vi "Main.vi"(0 "Operation":string(combo)="Add", 1 "Delete":bool, 5 "Add":bool, 7 "Load":bool, 9 "Save":bool, 11 "Error In":errorcluster, 12 "Tree":string(tree)) -> (15 "Error Out":errorcluster)   [LabVIEW 2021, in "Calculator.lvlib"]
doc: "This VI acts as a calculator , which has four child classes with the overriding methods and seperate UI VIs for each class which is opened in subpanel when the particular instance is selected. Also the class data is stored in XML file and it can be loaded when required."
uses:
  Calculator.lvlib
  Controls/Queue Operations.ctl
  Classes/NumericOperation/NumericOperation.lvclass
  Controls/Data Cluster.ctl
  Controls/Class Data.ctl
  Controls/User Event Operations.ctl
  <vilib>/Utility/xml.llb/Write to XML File(string).vi
  <vilib>/Utility/xml.llb/Read From XML File(array).vi
panel:
  in  "Help Button":bool
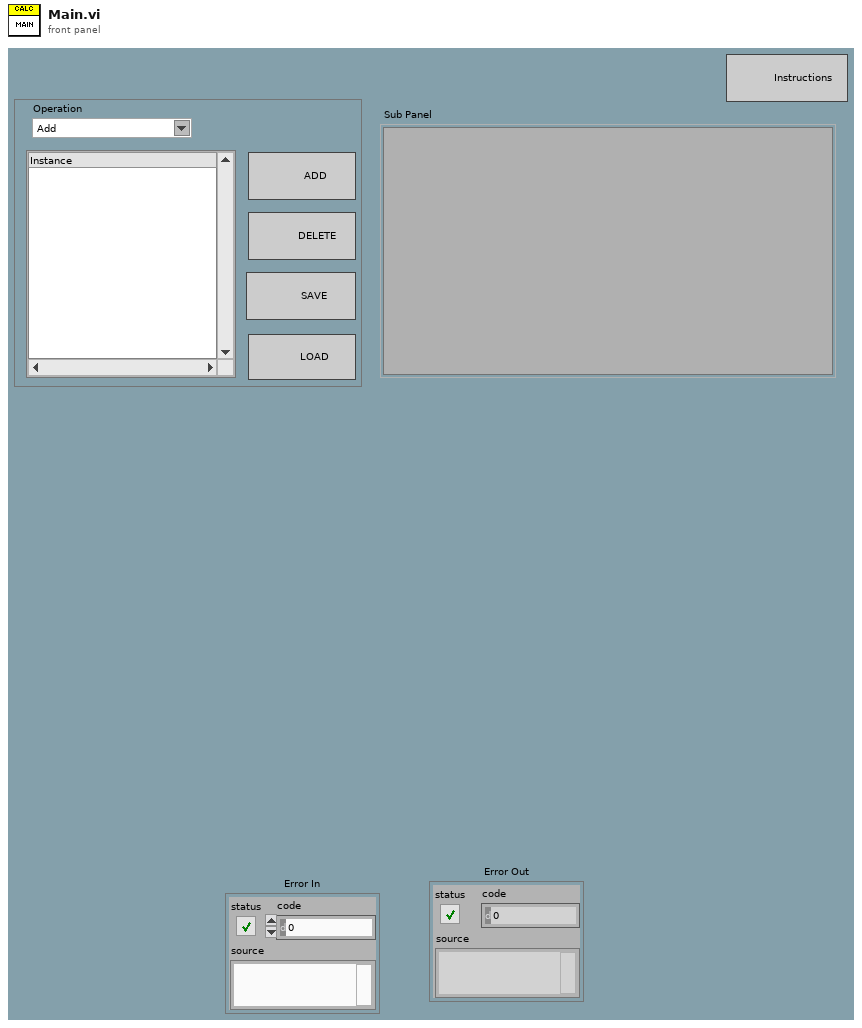
[diagram p1: front panel]
types:
  T1 = typedef "Calculator.lvlib/User Event Operations.ctl" = enum16{"Obtain", "Generate", "Release"}
  T2 = typedef "Calculator.lvlib/Queue Operations.ctl" = enum16{"Create", "Enqueue", "EnqueueN", "Enqueue at top", "Dequeue", "Flush", "Release"}
  T3 = typedef "Calculator.lvlib/Data Cluster.ctl" = cluster{"A":dbl, "B":dbl, "C":dbl, "NumericOperation.lvclass":refnum<class "NumericOperation.lvclass">, "generic class reference":refnum<class "NumericOperation.lvclass">, "Operation":string, "Active Tag":string, "Path":path, "VI Refnum":refnum<vi>, "Class Data":refnum<class "NumericOperation.lvclass">, "DataArray":T4[], "FilePath":path, "Class Name":string, "Data Value Reference Out":refnum<data-value>}
  T4 = typedef "Calculator.lvlib/Class Data.ctl" = cluster{"Class Data":refnum<class "NumericOperation.lvclass">, "String":string}
  T5 = typedef "LVPoint32TypeDef.ctl" = cluster{"Horizontal":i32, "Vertical":i32}
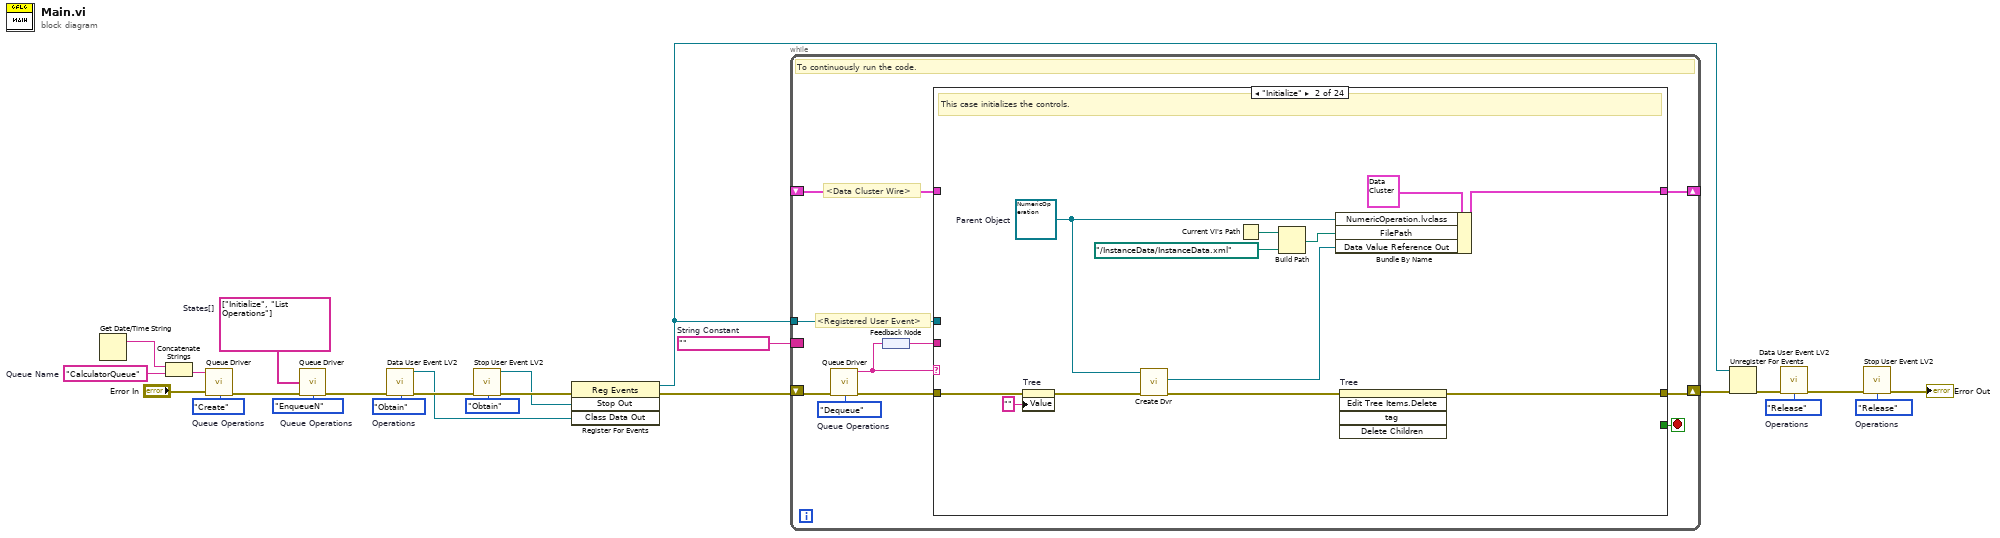
[diagram p0: block diagram]
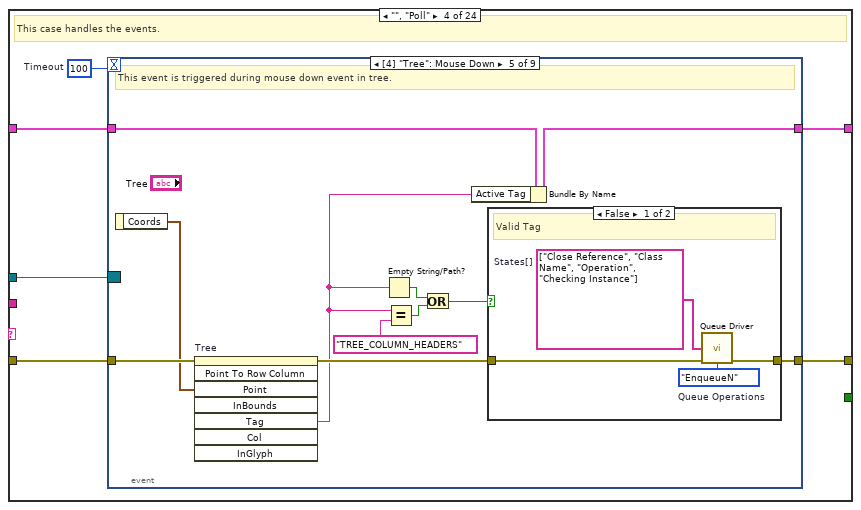
[diagram p4: hidden frame]
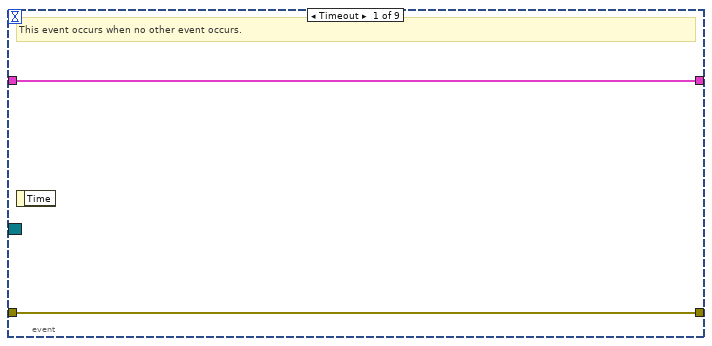
[diagram p5: hidden frame]
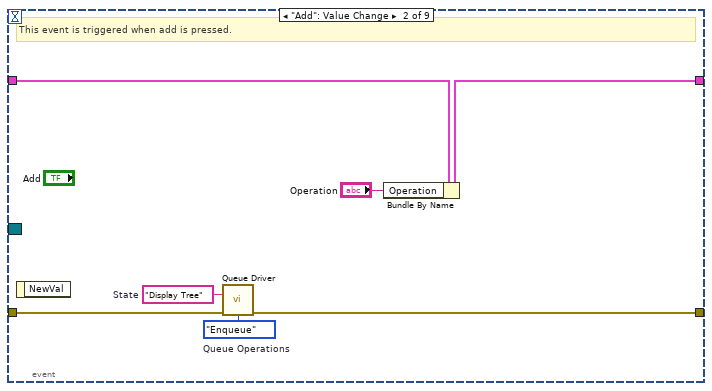
[diagram p6: hidden frame]
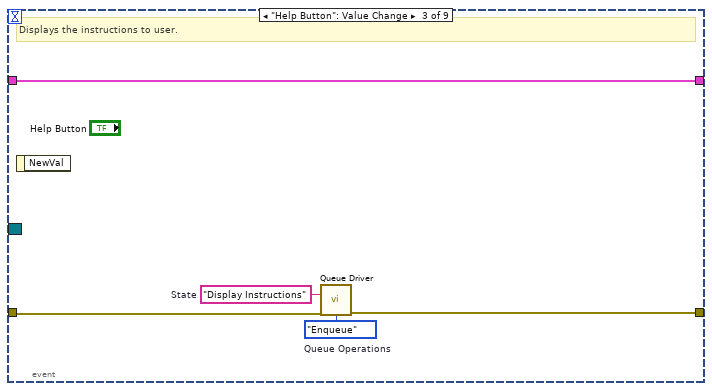
[diagram p7: hidden frame]
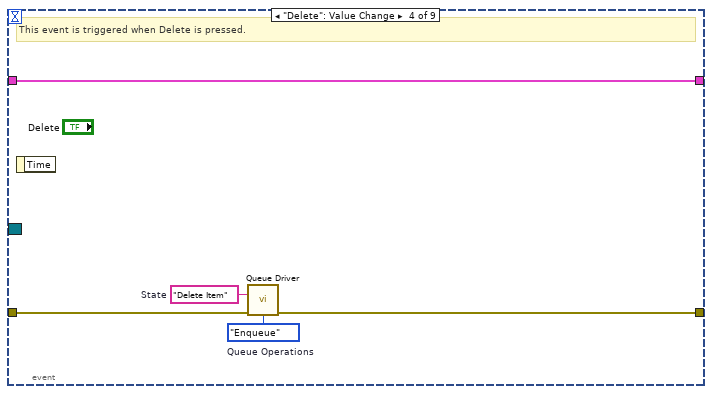
[diagram p8: hidden frame]
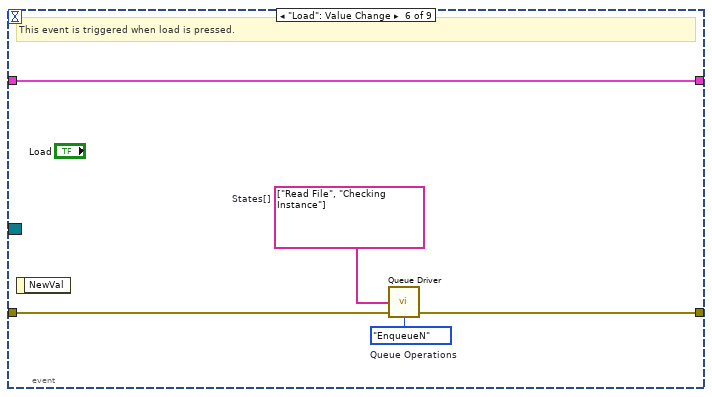
[diagram p10: hidden frame]
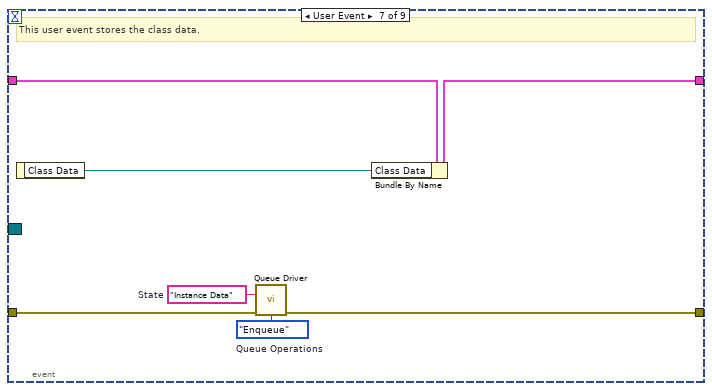
[diagram p11: hidden frame]
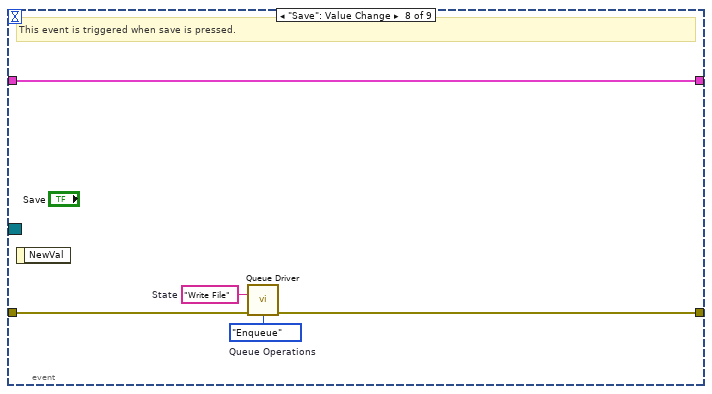
[diagram p12: hidden frame]
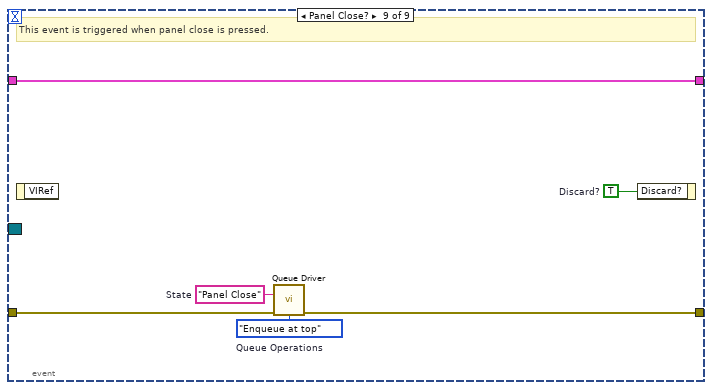
[diagram p13: hidden frame]
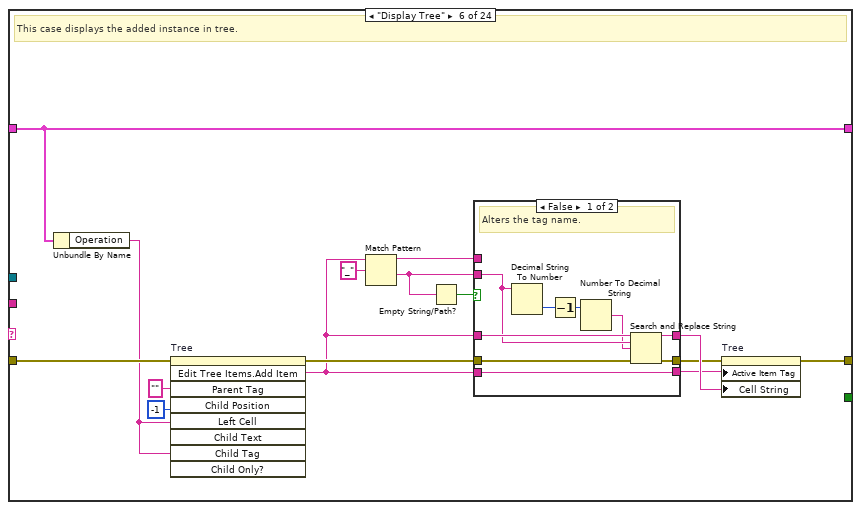
[diagram p15: hidden frame]
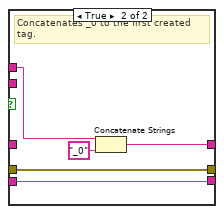
[diagram p16: hidden frame]
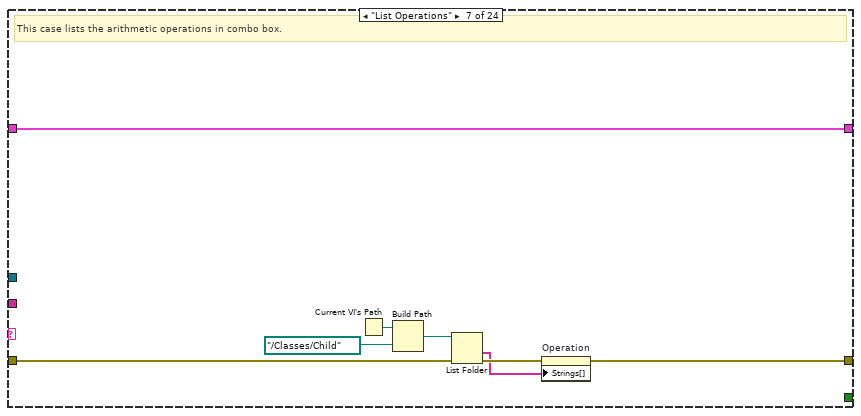
[diagram p17: hidden frame]
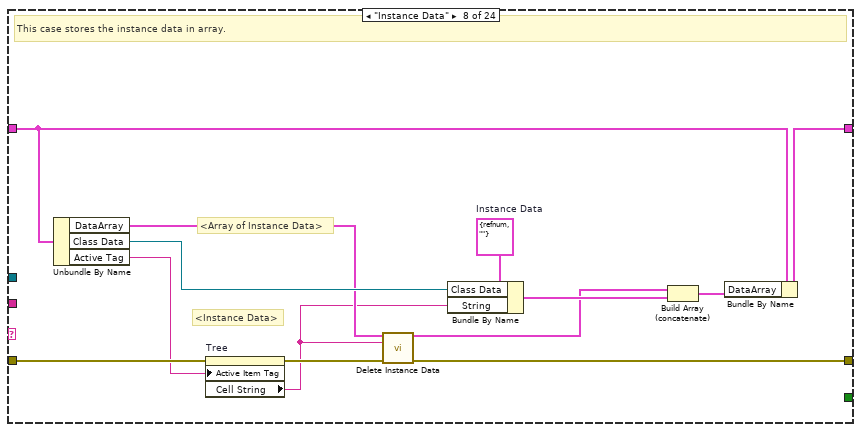
[diagram p18: hidden frame]
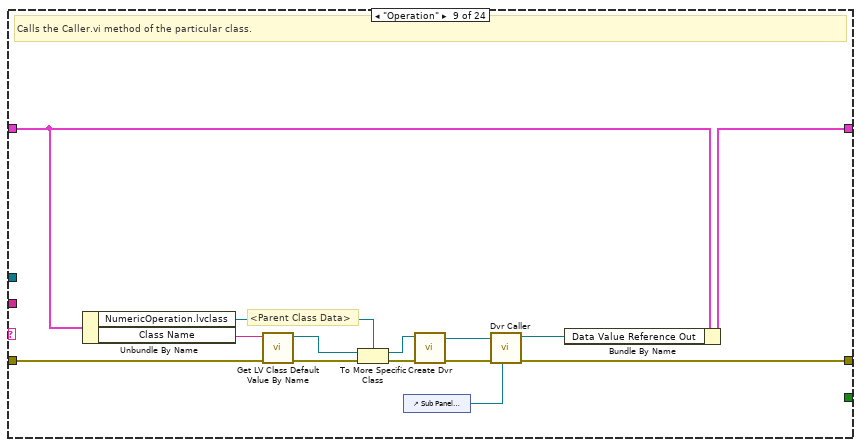
[diagram p19: hidden frame]
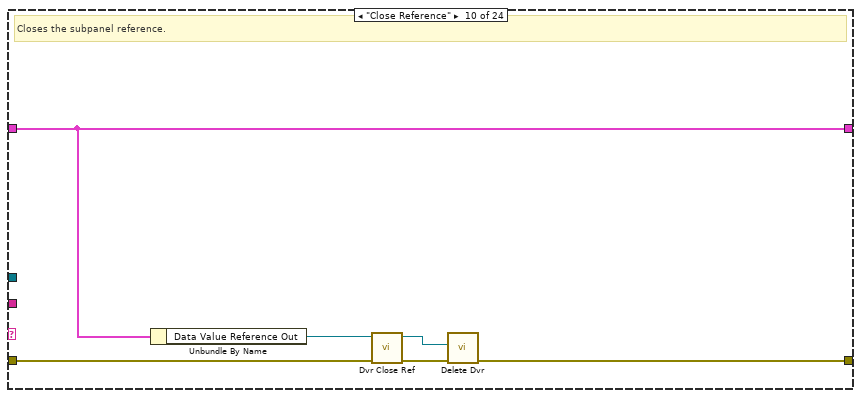
[diagram p20: hidden frame]
diagram:
  w1 = string[] ["Initialize", "List Operations"]  # States[]
  w2 = ""  # String Constant
  w3 = User_Event_Operations."Release"  # Operations
  w4 = User_Event_Operations."Release"  # Operations
  w11 = User_Event_Operations."Obtain"  # Operations
  w21 = Queue_Operations."EnqueueN"  # Queue Operations
  w19 = "CalculatorQueue"  # Queue Name
  w23 = Queue_Operations."Create"  # Queue Operations
  n1 = Get Date/Time String() -> (date string=w20:string)  [unwired: 3 in, 1 out]
  n2 = Concatenate Strings(w20, w19) -> (w18:string)
  n3 = call "Queue Driver.vi"("Queue Name"=w18, "Error In"="Error In", "Queue Operations"=w23) -> ("Error Out"=w22:errorcluster)  [unwired: 11 in, 1 out]
  n4 = call "Queue Driver.vi"("States[]"=w1, "Error In"=w22, "Queue Operations"=w21) -> ("Error Out"=w13:errorcluster)  [unwired: 11 in, 1 out]
  n5 = call "Data User Event LV2.vi"("Error In"=w13, "Operations"=w11) -> ("Class Data Out"=w8:refnum<user-event>, "Error Out"=w14:errorcluster)  [unwired: 12 in]
  n6 = call "Stop User Event LV2.vi"("Error In"=w14, "Operations"=User_Event_Operations."Obtain") -> ("Stop Out"=w9:refnum<user-event>, "Error Out"=w12:errorcluster)  [unwired: 12 in]
  n7 = register-events(error in=w12, w9, w8) -> (reference out=w15:refnum<event-registration>, error out=w17:errorcluster)  [unwired: 1 in]
  n8 = while {
    shift-right: [w32] -> _
    shift-left: _ -> [w33]
    shift-right: [w29] -> w16
    shift-left: w17 -> [w30]
    border: w2 -> [_]
    tunnel: w15 -> [w25]
    stop <- w26 stop-if-true
    w34 = Queue_Operations."Dequeue"  # Queue Operations
    # "<Registered User Event>"
    # "<Data Cluster Wire>"
    # "To continuously run the code."
    n9 = call "Queue Driver.vi"("Error In"=w30, "Queue Operations"=w34) -> ("Dequeued Element"=w28:string, "Error Out"=w31:errorcluster)  [unwired: 12 in]
    n10 = feedback-in #1(w28) -> ()
    n11 = feedback #1() -> (w27:string)
    n12 = case shown="\"Initialize\"" w28 {
      tunnel: w33 -> [w36 _ w50 w55 w116 w122 w153 w165 w175 w186 w190 w218 w226 w247 w256 w262 w276 w292 w297 w304 w307 w309 w312 w329]
      tunnel: [w36 w48 w50 w54 w116 w122 w153 w164 w177 w186 w188 w217 w226 w247 w256 w262 w275 w292 w297 w304 w307 w309 w312 w329] -> w32
      tunnel: w31 -> [w35 w39 w49 w53 w115 w131 w149 w166 w176 w185 w194 w216 w221 w246 w255 w259 w280 w291 w296 w303 w306 w308 w311 w328]
      tunnel: [w35 w46 w49 w52 w115 w126 w152 w157 w171 w182 w195 w216 w224 w245 w255 w260 w273 w291 w299 w303 w306 w308 w314 w328] -> w29
      tunnel: w27 -> [_ _ _ _ _ _ _ _ _ _ _ _ _ _ _ _ _ _ _ _ _ _ w321 _]
      tunnel: [_ _ _ _ _ _ _ _ _ _ _ _ _ _ _ _ _ _ w298 _ _ _ _ _] -> w26
      tunnel: w25 -> [_ _ _ w51 _ _ _ _ _ _ _ _ _ _ _ _ _ _ _ _ _ _ _ _]
      frame "/******** Initializing********/" {
        # "Splitter case for initialization."
      }
      frame "Initialize" {
        w41 = refnum<class "NumericOperation.lvclass"> refnum  # Parent Object
        # "This case initializes the controls."
        n13 = property on="Tree" class="Tree (strict)"(error in=w39, "Value"="" ("Tree")) -> (error out=w38:errorcluster)  [unwired: 1 in, 1 out]
        n14 = call "Create Dvr.vi"("Error In"=w38, "NumericOperation in"=w41) -> ("Error Out"=w42:errorcluster, "Data Value Reference"=w40:refnum<data-value>)  [unwired: 7 in, 1 out]
        n15 = Current VI's Path() -> (path=w45:path)
        n16 = Build Path(base path=w45, name or relative path=path "../InstanceData/InstanceData.xml") -> (appended path=w47:path)
        n17 = Bundle By Name(cluster=T3 {"A"=0.0, "B"=0.0, "C"=0.0, "NumericOperation.lvclass"=refnum, "generic class reference"=refnum, "Operation"="", "Active Tag"="", "Path"=path "", "VI Refnum"=refnum, "Class Data"=refnum, "DataArray"=[], "FilePath"=path "", "Class Name"="", "Data Value Reference Out"=refnum}, "NumericOperation.lvclass"=w41, "FilePath"=w47, "Data Value Reference Out"=w40) -> (w48:T3)
        n18 = invoke on="Tree" class="Tree (strict)" method="Edit Tree Items.Delete"(error in=w42) -> (error out=w46:errorcluster)  [unwired: 4 in, 4 out]
      }
      frame "/******** Poll ********/" {
        # "Splitter case for poll."
      }
      frame "", "Poll" {
        w56 = 100  # Timeout
        # "This case handles the events."
        n19 = event shown="[4] \"Tree\": Mouse Down" {
          selector: w51 -> [_ _ _ _ _ _ _ _ _]
          dyn-events: _ -> [_ _ _ _ _ _ _ _ _]
          timeout: w56 -> [_ _ _ _ _ _ _ _ _]
          tunnel: w55 -> [w58 w61 w66 w71 w84 w96 w103 w108 w111]
          tunnel: [w58 w60 w66 w71 w83 w96 w101 w108 w111] -> w54
          tunnel: w53 -> [w57 w65 w70 w75 w86 w94 w99 w107 w114]
          tunnel: [w57 w64 w69 w74 w81 w95 w100 w106 w113] -> w52
          event Timeout {
            # "This event occurs when no other event occurs."
            n20 = event-data() -> ()  [unwired: 1 in, 1 out]
          }
          event "Add": Value Change {
            w62 = "Display Tree"  # State
            w63 = Queue_Operations."Enqueue"  # Queue Operations
            # "This event is triggered when add is pressed."
            n21 = event-data() -> ()  [unwired: 1 in, 1 out]
            n22 = call "Queue Driver.vi"("State"=w62, "Error In"=w65, "Queue Operations"=w63) -> ("Error Out"=w64:errorcluster)  [unwired: 11 in, 1 out]
            n23 = Bundle By Name(cluster=w61, "Operation"="Operation") -> (w60:T3)
          }
          event "Help Button": Value Change {
            w67 = "Display Instructions"  # State
            w68 = Queue_Operations."Enqueue"  # Queue Operations
            # "Displays the instructions to user."
            n24 = event-data() -> ()  [unwired: 1 in, 1 out]
            n25 = call "Queue Driver.vi"("State"=w67, "Error In"=w70, "Queue Operations"=w68) -> ("Error Out"=w69:errorcluster)  [unwired: 11 in, 1 out]
          }
          event "Delete": Value Change {
            w72 = "Delete Item"  # State
            w73 = Queue_Operations."Enqueue"  # Queue Operations
            # "This event is triggered when Delete is pressed."
            n26 = event-data() -> ()  [unwired: 1 in, 1 out]
            n27 = call "Queue Driver.vi"("State"=w72, "Error In"=w75, "Queue Operations"=w73) -> ("Error Out"=w74:errorcluster)  [unwired: 11 in, 1 out]
          }
          event "Tree": Mouse Down {
            # "This event is triggered during mouse down event in tree."
            n28 = event-data() -> ("Coords"=w85:T5)  [unwired: 1 in]
            n29 = invoke on="Tree" class="Tree (strict)" method="Point To Row Column"(error in=w86, "Point"=w85) -> (error out=w82:errorcluster, "Tag"=w80:string)  [unwired: 6 in, 6 out]
            n30 = Empty String/Path?(string/path=w80) -> (empty?=w77:bool)
            n31 = Equal?(x=w80, y="TREE_COLUMN_HEADERS") -> (x = y?=w78:bool)
            n32 = Or(x=w77, y=w78) -> (x .or. y?=w76:bool)
            n33 = Bundle By Name(cluster=w84, "Active Tag"=w80) -> (w83:T3)
            n34 = case shown="False" w76 {
              tunnel: w82 -> [w90 w91]
              tunnel: [w89 w91] -> w81
              frame False {
                w87 = string[] ["Close Reference", "Class Name", "Operation", "Checking Instance"]  # States[]
                w88 = Queue_Operations."EnqueueN"  # Queue Operations
                # "Valid Tag"
                n35 = call "Queue Driver.vi"("States[]"=w87, "Error In"=w90, "Queue Operations"=w88) -> ("Error Out"=w89:errorcluster)  [unwired: 11 in, 1 out]
              }
              frame True {
                # "Invalid Tag"
              }
            }
          }
          event "Load": Value Change {
            w92 = string[] ["Read File", "Checking Instance"]  # States[]
            w93 = Queue_Operations."EnqueueN"  # Queue Operations
            # "This event is triggered when load is pressed."
            n36 = event-data() -> ()  [unwired: 1 in, 1 out]
            n37 = call "Queue Driver.vi"("States[]"=w92, "Error In"=w94, "Queue Operations"=w93) -> ("Error Out"=w95:errorcluster)  [unwired: 11 in, 1 out]
          }
          event User Event {
            w97 = "Instance Data"  # State
            w98 = Queue_Operations."Enqueue"  # Queue Operations
            # "This user event stores the class data."
            n38 = event-data() -> ("Class Data"=w102:refnum<class "NumericOperation.lvclass">)  [unwired: 1 in]
            n39 = call "Queue Driver.vi"("State"=w97, "Error In"=w99, "Queue Operations"=w98) -> ("Error Out"=w100:errorcluster)  [unwired: 11 in, 1 out]
            n40 = Bundle By Name(cluster=w103, "Class Data"=w102) -> (w101:T3)
          }
          event "Save": Value Change {
            w104 = "Write File"  # State
            w105 = Queue_Operations."Enqueue"  # Queue Operations
            # "This event is triggered when save is pressed."
            n41 = event-data() -> ()  [unwired: 1 in, 1 out]
            n42 = call "Queue Driver.vi"("State"=w104, "Error In"=w107, "Queue Operations"=w105) -> ("Error Out"=w106:errorcluster)  [unwired: 11 in, 1 out]
          }
          event Panel Close? {
            w110 = Queue_Operations."Enqueue at top"  # Queue Operations
            w112 = "Panel Close"  # State
            w109 = TRUE  # Discard?
            # "This event is triggered when panel close is pressed."
            n43 = event-data() -> ()  [unwired: 1 in, 1 out]
            n44 = call "Queue Driver.vi"("State"=w112, "Error In"=w114, "Queue Operations"=w110) -> ("Error Out"=w113:errorcluster)  [unwired: 11 in, 1 out]
            n45 = event-data("Discard?"=w109) -> ()  [unwired: 1 in, 1 out]
          }
        }
      }
      frame "/******** Functionalities ********/" {
        # "Splitter case for functionalities."
      }
      frame "Display Tree" {
        # "This case displays the added instance in tree."
        n46 = Unbundle By Name(w122) -> ("Operation"=w121:string)
        n47 = invoke on="Tree" class="Tree (strict)" method="Edit Tree Items.Add Item"(error in=w131, "Parent Tag"="", "Child Position"=-1, "Left Cell"=w121, "Child Tag"=w121) -> (error out=w120:errorcluster, "Edit Tree Items:Add Item"=w118:string)  [unwired: 4 in, 7 out]
        n48 = Match Pattern(string=w118, regular expression="_") -> (before substring=w127:string, after substring=w123:string)  [unwired: 1 in, 2 out]
        n49 = Empty String/Path?(string/path=w123) -> (empty?=w124:bool)
        n50 = case shown="False" w124 {
          tunnel: [w137 w144] -> w125
          tunnel: w127 -> [_ w143]
          tunnel: w123 -> [w138 _]
          tunnel: w118 -> [w139 _]
          tunnel: w120 -> [w134 w142]
          tunnel: [w133 w142] -> w119
          tunnel: [w132 w141] -> w117
          tunnel: w118 -> [w132 w141]
          frame False {
            # "Alters the tag name."
            n51 = Decimal String To Number(string=w138) -> (number=w136:i32)  [unwired: 2 in, 1 out]
            n52 = Decrement(x=w136) -> (x-1=w140:i32)
            n53 = Number To Decimal String(number=w140) -> (decimal integer string=w135:string)  [unwired: 1 in]
            n54 = Search and Replace String(input string=w139, search string=w138, replace string=w135, error in=w134) -> (result string=w137:string, error out=w133:errorcluster)  [unwired: 4 in, 2 out]
          }
          frame True {
            # "Concatenates _0 to the first created tag."
            n55 = Concatenate Strings(w143, "_0" ("string")) -> (w144:string)
          }
        }
        n56 = property on="Tree" class="Tree (strict)"(error in=w119, "Active Item Tag"=w117, "Cell String"=w125) -> (error out=w126:errorcluster)  [unwired: 1 in, 1 out]
      }
      frame "List Operations" {
        # "This case lists the arithmetic operations in combo box."
        n57 = Current VI's Path() -> (path=w151:path)
        n58 = Build Path(base path=w151, name or relative path=path "../Classes/Child") -> (appended path=w147:path)
        n59 = List Folder(path=w147, error in=w149) -> (folder names=w146:string[], error out=w148:errorcluster)  [unwired: 2 in, 2 out]
        n60 = property on="Operation" class="CmbBox"(error in=w148, "Strings[]"=w146) -> (error out=w152:errorcluster)  [unwired: 1 in, 1 out]
      }
      frame "Instance Data" {
        w162 = T4 {"Class Data"=refnum, "String"=""}  # Instance Data
        # "<Array of Instance Data>"
        # "<Instance Data>"
        # "This case stores the instance data in array."
        n61 = Unbundle By Name(w165) -> ("DataArray"=w156:T4[], "Class Data"=w161:refnum<class "NumericOperation.lvclass">, "Active Tag"=w163:string)
        n62 = property on="Tree" class="Tree (strict)"(error in=w166, "Active Item Tag"=w163) -> (error out=w158:errorcluster, "Cell String"=w155:string)  [unwired: 1 in, 1 out]
        n63 = call "Delete Instance Data.vi"("Data Array"=w156, "Cell String"=w155, "Error In"=w158) -> ("Data Array Out"=w154:T4[], "Error Out"=w157:errorcluster)  [unwired: 11 in]
        n64 = Bundle By Name(cluster=w162, "Class Data"=w161, "String"=w155) -> (w160:T4)
        n65 = Build Array (concatenate)(w154, w160) -> (w159:T4[])
        n66 = Bundle By Name(cluster=w165, "DataArray"=w159) -> (w164:T3)
      }
      frame "Operation" {
        # "<Parent Class Data>"
        # "Calls the Caller.vi method of the particular class."
        n67 = Unbundle By Name(w175) -> ("NumericOperation.lvclass"=w174:refnum<class "NumericOperation.lvclass">, "Class Name"=w178:string)
        n68 = call <vilib>:"Get LV Class Default Value By Name.vi"("error in (no error)"=w176, "class name"=w178) -> ("error out"=w179:errorcluster, "object"=w180:refnum<class>)  [unwired: 8 in]
        n69 = To More Specific Class(target class=w174, reference=w180, error in=w179) -> (specific class reference=w170:refnum<class "NumericOperation.lvclass">, error out=w172:errorcluster)
        n70 = control-ref of="Sub Panel Reference"() -> (w168:refnum<vi>)
        n71 = call "Create Dvr.vi"("Error In"=w172, "NumericOperation in"=w170) -> ("Error Out"=w173:errorcluster, "Data Value Reference"=w169:refnum<data-value>)  [unwired: 7 in, 1 out]
        n72 = call "Dvr Caller.vi"("Sub Panel"=w168, "Error In"=w173, "Data Value Reference In"=w169) -> ("Error Out"=w171:errorcluster, "Data Value Reference Out"=w167:refnum<data-value>)  [unwired: 7 in]
        n73 = Bundle By Name(cluster=w175, "Data Value Reference Out"=w167) -> (w177:T3)
      }
      frame "Close Reference" {
        # "Closes the subpanel reference."
        n74 = Unbundle By Name(w186) -> ("Data Value Reference Out"=w184:refnum<data-value>)
        n75 = call "Dvr Close Ref.vi"("Error In"=w185, "Data Value Reference In"=w184) -> ("Error Out"=w183:errorcluster, "Data Value Reference Out"=w181:refnum<data-value>)  [unwired: 8 in]
        n76 = call "Delete Dvr.vi"("Error In"=w183, "Data Value Reference"=w181) -> ("Error Out"=w182:errorcluster)  [unwired: 9 in]
      }
      frame "Delete Item" {
        # "Deletes the item from tree."
        n77 = property on="Tree" class="Tree (strict)"(error in=w194) -> (error out=w193:errorcluster, "Value"=w187:string)  [unwired: 1 in, 1 out]
        n78 = Unbundle By Name(w190) -> ("DataArray"=w191:T4[])
        n79 = Empty String/Path?(string/path=w187) -> (empty?=w192:bool)
        n80 = case shown="False" w192 {
          tunnel: [w205 w209] -> w195
          tunnel: w193 -> [w199 w209]
          tunnel: w191 -> [w202 w207]
          tunnel: [w201 w207] -> w189
          tunnel: w187 -> [w197 _]
          frame False {
            # "Valid Tag"
            n81 = property on="Tree" class="Tree (strict)"(error in=w199, "Active Item Tag"=w197) -> (error out=w198:errorcluster, "Cell String"=w196:string)  [unwired: 1 in, 1 out]
            n82 = invoke on="Tree" class="Tree (strict)" method="Edit Tree Items.Delete"(error in=w198, "tag"=w197) -> (error out=w200:errorcluster)  [unwired: 3 in, 4 out]
            n83 = call "Delete Instance Data.vi"("Data Array"=w202, "Cell String"=w196, "Error In"=w200) -> ("Data Array Out"=w201:T4[], "Error Out"=w203:errorcluster)  [unwired: 11 in]
            n84 = invoke on="Sub Panel" class="SubPnl" method="Remove VI"(error in=w203) -> (error out=w206:errorcluster)  [unwired: 2 in, 2 out]
            n85 = property on="Tree" class="Tree (strict)"(error in=w206, "Value"="" ("Tree")) -> (error out=w205:errorcluster)  [unwired: 1 in, 1 out]
          }
          frame True {
            # "No item is selected."
            n86 = One Button Dialog(message="Select Instance to Delete") -> ()  [unwired: 1 in, 1 out]
          }
        }
        n87 = Bundle By Name(cluster=w190, "DataArray"=w189) -> (w188:T3)
      }
      frame "Class Name" {
        # "Gives the class name of the active instance."
        n88 = Unbundle By Name(w218) -> ("Active Tag"=w215:string)
        n89 = Match Pattern(string=w215, regular expression="_") -> (before substring=w213:string)  [unwired: 1 in, 3 out]
        n90 = Concatenate Strings("Calculator.lvlib:" ("string"), w213, ".lvclass" ("string")) -> (w211:string)
        n91 = Bundle By Name(cluster=w218, "Class Name"=w211) -> (w217:T3)
      }
      frame "Checking Instance" {
        # "Gives the recent data of active instance that is stored in array."
        n92 = Unbundle By Name(w226) -> ("DataArray"=w225:T4[], "Active Tag"=w222:string)
        n93 = property on="Tree" class="Tree (strict)"(error in=w221) -> (error out=w220:errorcluster, "Value"=w219:string)  [unwired: 1 in, 1 out]
        n94 = Empty String/Path?(string/path=w219) -> (empty?=w223:bool)
        n95 = case shown="False" w223 {
          tunnel: w222 -> [w235 _]
          tunnel: w225 -> [w233 _]
          tunnel: [w230 w243] -> w224
          tunnel: w220 -> [w227 w243]
          frame False {
            w228 = User_Event_Operations."Generate"  # Operations
            # "valid tag"
            n96 = Reverse 1D Array(array=w233) -> (reversed array=w232:T4[])
            n97 = property on="Tree" class="Tree (strict)"(error in=w227, "Active Item Tag"=w235) -> (error out=w236:errorcluster, "Cell String"=w234:string)  [unwired: 1 in, 1 out]
            n98 = for {
              tunnel: w234 -> [w241]
              tunnel: w232 -> [w239] mode=indexing
              tunnel: [w238] -> w229 if=w237
              shift-right: [w240] -> w231
              shift-left: w236 -> [w240]
              stop <- w237 stop-if-true
              # "Search for the recent instance from array"
              n99 = Unbundle By Name(w239) -> ("Class Data"=w238:refnum<class "NumericOperation.lvclass">, "String"=w242:string)
              n100 = Equal?(x=w242, y=w241) -> (x = y?=w237:bool)
            }
            n101 = call "Data User Event LV2.vi"("Class Data"=w229, "Error In"=w231, "Operations"=w228) -> ("Error Out"=w230:errorcluster)  [unwired: 11 in, 1 out]
          }
          frame True {
            # "Invalid Tag"
          }
        }
      }
      frame "Load Instance Data" {
        # "Loads the saved instance data in tree on new run of the VI."
        n102 = Unbundle By Name(w247) -> ("DataArray"=w244:T4[])
        n103 = for {
          shift-right: [w249] -> w245
          shift-left: w246 -> [w254]
          tunnel: w244 -> [w252] mode=indexing
          # "Populates the saved instance to tree"
          n104 = Unbundle By Name(w252) -> ("String"=w248:string)
          n105 = Match Pattern(string=w248, regular expression="_") -> (before substring=w250:string)  [unwired: 1 in, 3 out]
          n106 = invoke on="Tree" class="Tree (strict)" method="Edit Tree Items.Add Item"(error in=w254, "Parent Tag"="", "Left Cell"=w248, "Child Tag"=w250) -> (error out=w249:errorcluster)  [unwired: 5 in, 8 out]
        }
      }
      frame "/******** File Operations ********/" {
        # "Splitter case for File Operations."
      }
      frame "Write File" {
        # "Flattens the class data and write it to the XML file."
        n107 = Unbundle By Name(w262) -> ("FilePath"=w261:path, "DataArray"=w258:T4[])
        n108 = Empty Array?(array=w258) -> (empty?=w257:bool)
        n109 = case shown="False" w257 {
          tunnel: w261 -> [w267 _]
          tunnel: [w266 w268] -> w260
          tunnel: w259 -> [w265 w268]
          tunnel: w258 -> [w263 _]
          frame False {
            # "Stores Data"
            n110 = Flatten To XML(6:w263) -> (2:w264:string)
            n111 = call-poly <vilib>:"Write to XML File.vi"("error in (no error)"=w265, "XML Input"=w264, "XML File Path"=w267) -> ("error out"=w266:errorcluster)  [unwired: 6 in, 2 out]
          }
          frame True {
            # "Empty Array."
          }
        }
      }
      frame "Read File" {
        # "Reads the stored data from XML file and unflattens the data to store in array."
        n112 = Unbundle By Name(w276) -> ("FilePath"=w279:path)
        n113 = call-poly <vilib>:"Read From XML File.vi"("error in (no error)"=w280, "XML File Path"=w279) -> ("error out"=w278:errorcluster, "XML Elements"=w277:string[])  [unwired: 7 in, 1 out]
        n114 = for {
          shift-right: [w289] -> w272
          shift-left: w278 -> [w290]
          tunnel: w277 -> [w287] mode=indexing
          tunnel: [w288] -> w274 mode=concatenating
          w286 = T4[] []  # Array of Instance Data
          # "Unflattens the data."
          n115 = Unflatten From XML(xml string=w287, type=w286, error in (no error)=w290) -> (value=w288:T4[], error out=w289:errorcluster)
        }
        n116 = Bundle By Name(cluster=w276, "DataArray"=w274) -> (w275:T3)
        n117 = property on="Tree" class="Tree (strict)"(error in=w272) -> (error out=w271:errorcluster, "DispItems"=w270:string[])  [unwired: 1 in, 1 out]
        n118 = Empty Array?(array=w270) -> (empty?=w269:bool)
        n119 = case shown="True" w269 {
          tunnel: [w281 w285] -> w273
          tunnel: w271 -> [w281 w282]
          frame False {
            # "Tree is not empty."
          }
          frame True {
            # "Tree is empty"
            n120 = call "Queue Driver.vi"("State"="Load Instance Data", "Error In"=w282, "Queue Operations"=Queue_Operations."Enqueue") -> ("Error Out"=w285:errorcluster)  [unwired: 11 in, 1 out]
          }
        }
      }
      frame "/******** Panel Close ********/" {
        # "Splitter case for Panel Close."
      }
      frame "Panel Close" {
        w293 = TRUE  # Stop?
        w294 = User_Event_Operations."Generate"  # Operations
        w298 = TRUE  # Exit?
        w301 = Queue_Operations."Release"  # Queue Operations
        w302 = Queue_Operations."Flush"  # Queue Operations
        # "Stops the running VI ."
        n121 = call "Stop User Event LV2.vi"("Stop"=w293, "Error In"=w296, "Operations"=w294) -> ("Error Out"=w295:errorcluster)  [unwired: 11 in, 1 out]
        n122 = call "Queue Driver.vi"("Error In"=w295, "Queue Operations"=w302) -> ("Error Out"=w300:errorcluster)  [unwired: 12 in, 1 out]
        n123 = call "Queue Driver.vi"("Error In"=w300, "Queue Operations"=w301) -> ("Error Out"=w299:errorcluster)  [unwired: 12 in, 1 out]
      }
      frame "/******* Display Instruction ********/" {
        # "Splitter case for instruction display."
      }
      frame "Display Instructions" {
        # "Displays the instructions to user."
        n124 = One Button Dialog(message="INSTRUCTIONS :\n\n1. Select the Operation from the combo box.\n2. Press ADD to add the instance in tree.\n3. Click the added instance in tree and it opens in the subpanel.\n4. Enter the inputs and press calculate.\n5. Press SAVE to save the data in XML file after calculating for a particular instance.\n6. Press LOAD to load the saved data of instances from XML file.\n7. Select the instance to delete and press DELETE to delete that particular instance.\n") -> ()  [unwired: 1 in, 1 out]
      }
      frame "/******** Error Handling ********/" {
        # "Splitter case for Error Handling"
      }
      frame "Error" {
        # "This case handles the error."
        n125 = Unbundle By Name(w311) -> ("code"=w320:i32, "source"=w319:string)
        n126 = call <vilib>:"Clear Errors.vi"("error in (no error)"=w311) -> ("error out"=w310:errorcluster)  [unwired: 5 in, 1 out]
        n127 = Format Into String(format string="Error occurred in state \"%s\"!!\nError Code: %d\nError Source: %s\n\nDo you wish to continue?", error in=w310, w321, w320, w319) -> (resulting string=w316:string, error out=w315:errorcluster)  [unwired: 1 in]
        n128 = Two Button Dialog(message=w316, 1:"Exit" ("F button name (\"Cancel\")"), 2:"Continue" ("T button name (\"OK\")")) -> (T button?=w313:bool)
        n129 = case "Continue?" shown="False" w313 {
          tunnel: w315 -> [w326 w327]
          tunnel: [w325 w327] -> w314
          frame False {
            w324 = "Panel Close"  # State
            # "This case occurs when exit is pressed."
            n130 = call "Queue Driver.vi"("State"=w324, "Error In"=w326, "Queue Operations"=Queue_Operations."Enqueue") -> ("Error Out"=w325:errorcluster)  [unwired: 11 in, 1 out]
          }
          frame True {
            # "This case occurs when continue is pressed."
          }
        }
      }
      frame Default {
        # "Developer error."
      }
    }
  }
  n131 = Unregister For Events(event registration refnum=w15, error in=w16) -> (error out=w6:errorcluster)
  n132 = call "Data User Event LV2.vi"("Error In"=w6, "Operations"=w4) -> ("Error Out"=w7:errorcluster)  [unwired: 12 in, 1 out]
  n133 = call "Stop User Event LV2.vi"("Error In"=w7, "Operations"=w3) -> ("Error Out"=→"Error Out":errorcluster)  [unwired: 12 in, 1 out]
